vi "Write Signature Fields.vi"(8 "error in (no error)":errorcluster, 10 "Signature Fields":T1, 11 "Session in":refnum<class "Session.lvclass">) -> (0 "error out":errorcluster, 3 "Session out":refnum<class "Session.lvclass">)   [LabVIEW 2015, in "NI_Azure_Core.lvlib" / "Session.lvclass"]
uses:
  Session.lvclass
  Signature Fields.ctl
  Session.lvclass/Session.ctl
  NI_Azure_Core.lvlib
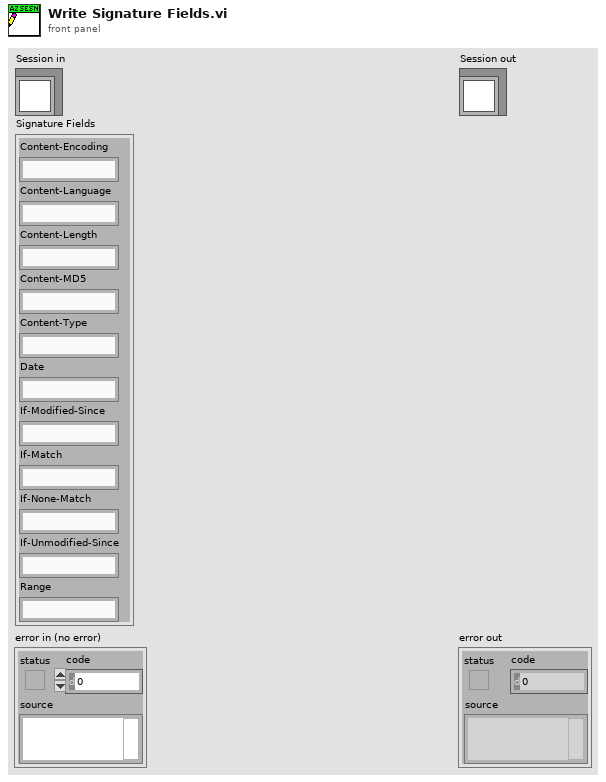
[diagram p1: front panel]
types:
  T1 = typedef "NI_Azure_Core.lvlib/Signature Fields.ctl" = cluster{"Content-Encoding":string, "Content-Language":string, "Content-Length":string, "Content-MD5":string, "Content-Type":string, "Date":string, "If-Modified-Since":string, "If-Match":string, "If-None-Match":string, "If-Unmodified-Since":string, "Range":string}
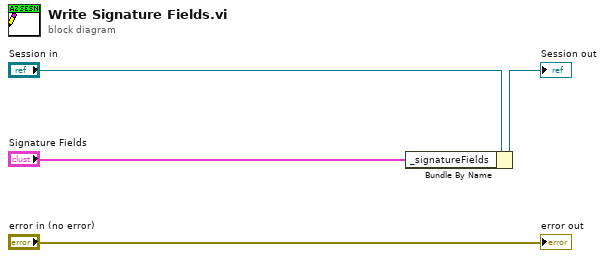
[diagram p0: block diagram]
diagram:
  n1 = Bundle By Name(cluster="Session in", "_signatureFields"="Signature Fields") -> (→"Session out":refnum<class "Session.lvclass">)
  "error out" <- "error in (no error)"
